vi "TCP.vi"() -> ()   [LabVIEW 2021]
panel:
  in  "stop":bool
  out "error out":errorcluster
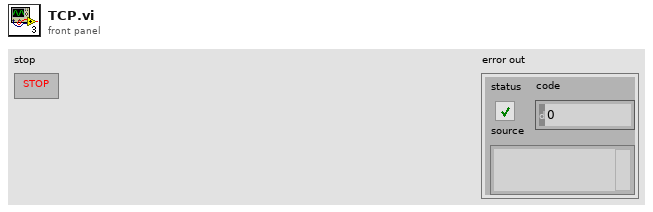
[diagram p1: front panel]
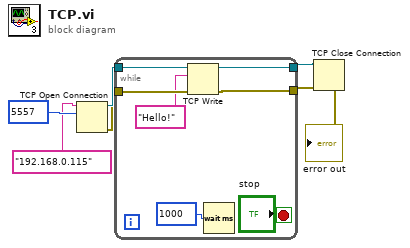
[diagram p0: block diagram]
diagram:
  n1 = TCP Open Connection(address="192.168.0.115", remote port or service name=u16 5557) -> (connection ID=w7:refnum<k5>, error out=w4:errorcluster)  [unwired: 3 in]
  n2 = while {
    tunnel: w7 -> [w14]
    tunnel: [w13] -> w6
    tunnel: [w12] -> w5
    tunnel: w4 -> [w11]
    stop <- "stop" stop-if-true
    n3 = TCP Write(connection ID=w14, data in="Hello!", error in (no error)=w11) -> (connection ID out=w13:refnum<k5>, error out=w12:errorcluster)  [unwired: 1 in, 1 out]
    n4 = Wait (ms)(milliseconds to wait=u32 1000) -> ()  [unwired: 1 out]
  }
  n5 = TCP Close Connection(connection ID=w6, error in (no error)=w5) -> (error out=→"error out":errorcluster)  [unwired: 1 in, 1 out]
